vi "Wechart Main.vi"() -> ()   [LabVIEW 2020]
panel:
  out "Reply":string
  in  "Send":bool
  in  "Open ID":string="o5NgY64UYqTYJlJ02s3ujBymuMNo"
  in  "Message":string
  # "https://mp.weixin.qq.com/debug/cgi-bin/sandboxinfo?action=showinfo&t=sandbox/index"
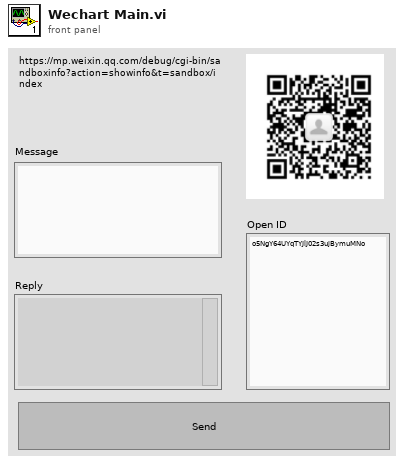
[diagram p1: front panel]
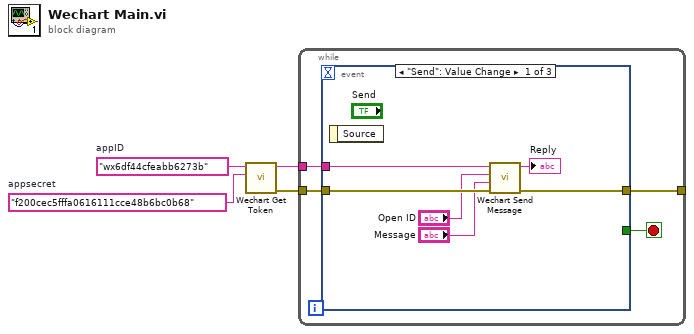
[diagram p0: block diagram]
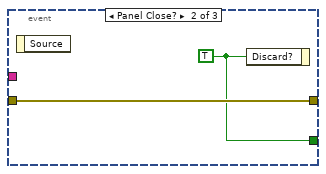
[diagram p2: hidden frame]
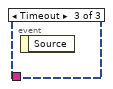
[diagram p3: hidden frame]
diagram:
  w3 = "f200cec5fffa0616111cce48b6bc0b68"  # appsecret
  w4 = "wx6df44cfeabb6273b"  # appID
  n1 = call "Wechart Get Token.vi"("appsecret"=w3, "appID"=w4) -> ("error out"=w2:errorcluster, "Token"=w1:string)  [unwired: 8 in]
  n2 = while {
    tunnel: w2 -> [w8]
    tunnel: w1 -> [w7]
    tunnel: [w6] -> _
    stop <- w5 stop-if-true
    n3 = event shown="[0] \"Send\": Value Change" {
      selector: _ -> [_ _ _]
      dyn-events: _ -> [_ _ _]
      timeout: _ -> [_ _ _]
      tunnel: w8 -> [w14 w16 _]
      tunnel: w7 -> [w13 _ _]
      tunnel: [w10 w16 _] -> w6
      tunnel: [_ w15 _] -> w5
      event "Send": Value Change {
        n4 = event-data() -> ()  [unwired: 1 in, 1 out]
        n5 = call "Wechart Send Message.vi"("error in"=w14, "content"="Message", "Open ID"="Open ID", "Token"=w13) -> ("error out"=w10:errorcluster, "Reply"=→"Reply":string)  [unwired: 6 in]
      }
      event Panel Close? {
        w15 = TRUE ("Discard?")
        n6 = event-data() -> ()  [unwired: 1 in, 1 out]
        n7 = event-data("Discard?"=w15) -> ()  [unwired: 1 in, 1 out]
      }
      event Timeout {
        n8 = event-data() -> ()  [unwired: 1 in, 1 out]
      }
    }
  }
